vi "OPCRead.vi"(1 "OPC URL":string) -> (0 "OPC Data":i32[](array[numeric]))   [LabVIEW 2013]
uses:
  GlobalVars.vi
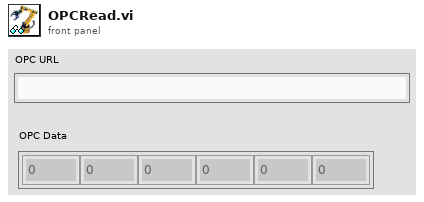
[diagram p1: front panel]
types:
  T1 = enum16{"Read", "Write", "ReadWrite", "BufferedRead", "BufferedReadWrite"}
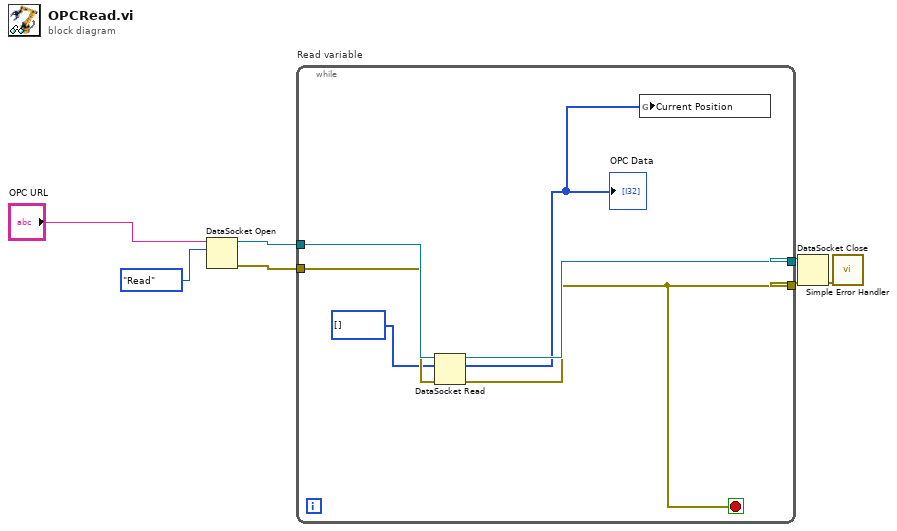
[diagram p0: block diagram]
diagram:
  n1 = DataSocket Open(10:T1."Read" ("mode"), 11:"OPC URL") -> (0:w5:errorcluster, 3:w7:refnum<k13>)  [unwired: 1 in, 1 out]
  n2 = while "Read variable" {
    tunnel: w7 -> [w13]
    tunnel: [w12] -> w6
    tunnel: w5 -> [w11]
    tunnel: [w10] -> w4
    stop <- w10 stop-if-true
    n3 = DataSocket Read(8:w11, 10:i32[] [] ("Array"), 11:w13) -> (0:w10:errorcluster, 2:w8:i32[], 3:w12:refnum<k13>)  [unwired: 6 out]
    "OPC Data" <- w8
    n4 = global write "GlobalVars.vi" "Current Position"(w8) -> ()
  }
  n5 = DataSocket Close(8:w4, 11:w6) -> (0:w3:errorcluster)  [unwired: 2 out]
  n6 = call <vilib>:"Simple Error Handler.vi"("error in (no error)"=w3) -> ()  [unwired: 4 in, 5 out]
